vi "AudioTest.Result Table to CSV Measurements File.vi"(8 "error in":errorcluster, 9 "Results Table":T1[](array[typedef]) caption="Results", 10 "Test Name":string, 11 "UUT Dir":path) -> (0 "error out":errorcluster, 3 "Out File":path)   [LabVIEW 2018]
uses:
  Common/Utils/Results/Result.Results Table Record.ctl
  <vilib>/KATE/Files/File Utils.lvlib
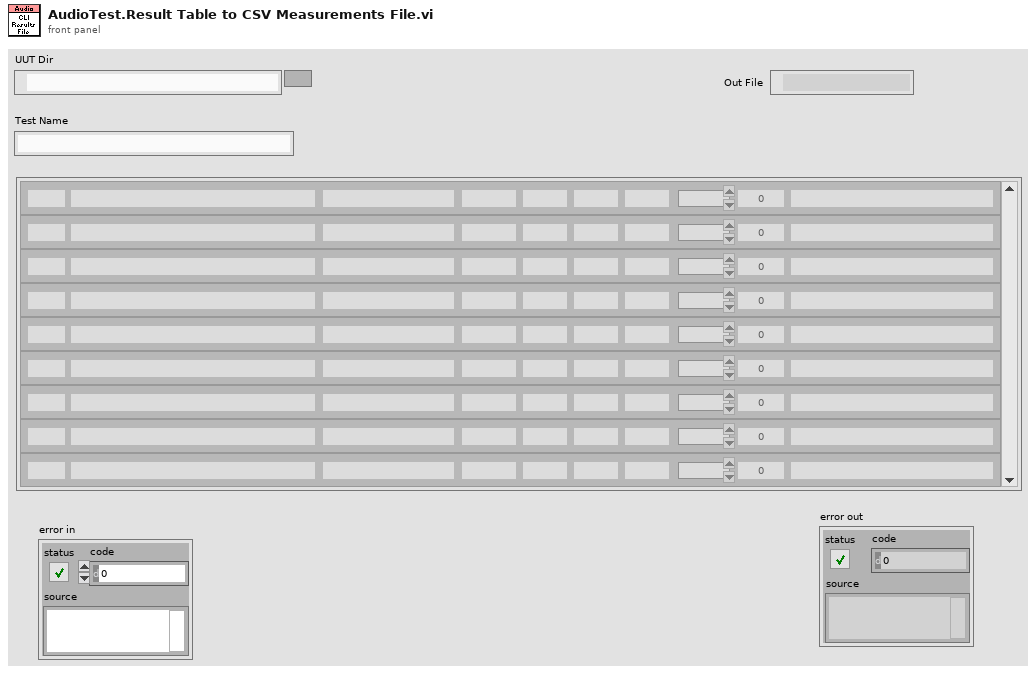
[diagram p1: front panel]
types:
  T1 = typedef "Result.Results Table Record.ctl" = cluster{"Cnt":i32, "Step":string, "Category":string, "Name":string, "Value":string, "Units":string, "LimType":string, "LL":string, "UL":string, "Status":string, "Status Color":u32, "Code":i32, "Desc":string}
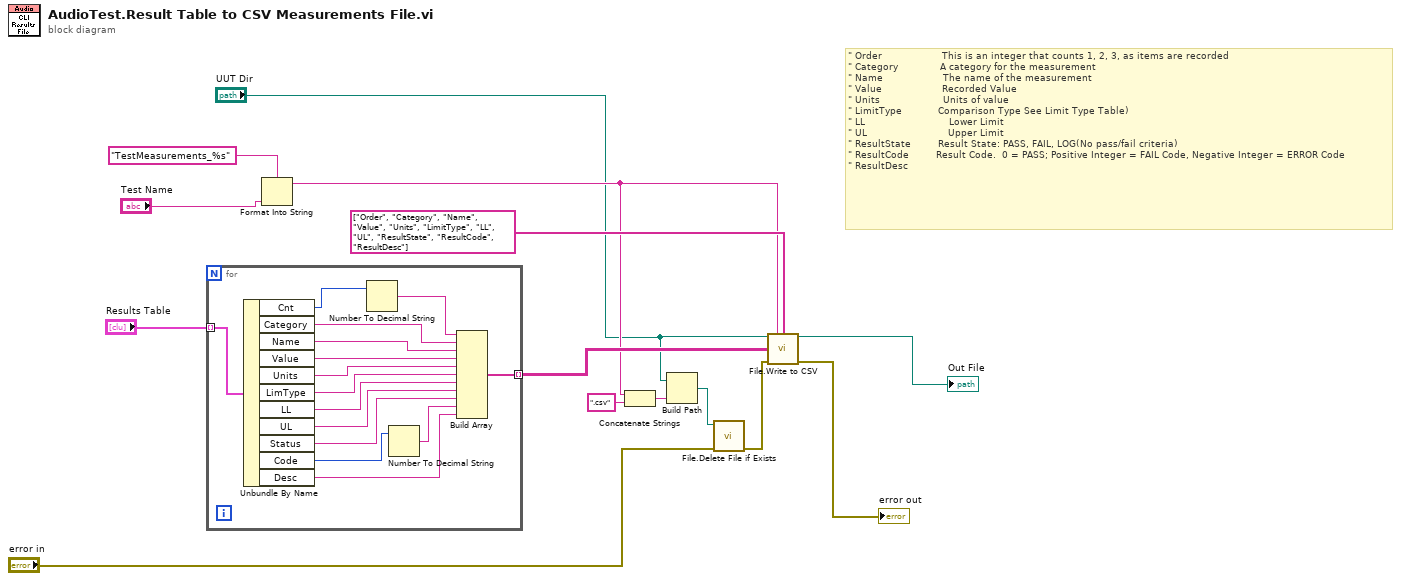
[diagram p0: block diagram]
diagram:
  # "\"\tOrder                    This is an integer that counts 1, 2, 3, as items are recorded\n\"\tCategory              A category for the measurement  \n\"\tName                    The name of the measurement\n\"\tValue                    Recorded Value\n\"\tUnits                     Units of value\n\"\tLimitType            Comparison Type See Limit Type Table) \n\"\tLL                            Lower Limit\n\"\tUL                           Upper Limit\n\"\tResultState         Result State: PASS, FAIL, LOG(No pass/fail criteria)\n\"\tResultCode         Result Code.  0 = PASS; Positive Integer = FAIL Code, Negative Integer = ERROR Code\n\"\tResultDesc"
  n1 = for {
    tunnel: "Results Table" -> [w29] mode=indexing
    tunnel: [w15] -> w10 mode=indexing
    n2 = Unbundle By Name(w29) -> ("Cnt"=w28:i32, "Category"=w25:string, "Name"=w24:string, "Value"=w23:string, "Units"=w22:string, "LimType"=w21:string, "LL"=w20:string, "UL"=w19:string, "Status"=w18:string, "Code"=w27:i32, "Desc"=w16:string)
    n3 = Number To Decimal String(number=w28) -> (decimal integer string=w26:string)  [unwired: 1 in]
    n4 = Number To Decimal String(number=w27) -> (decimal integer string=w17:string)  [unwired: 1 in]
    n5 = Build Array(w26, w25, w24, w23, w22, w21, w20, w19, w18, w17, w16) -> (w15:string[])
  }
  n6 = Format Into String(format string="TestMeasurements_%s", "Test Name") -> (resulting string=w6:string)  [unwired: 2 in, 1 out]
  n7 = Concatenate Strings(w6, ".csv" ("string")) -> (w5:string)
  n8 = Build Path(base path="UUT Dir", name or relative path=w5) -> (appended path=w1:path)
  n9 = call "File.Delete File if Exists.vi"("error in"="error in", "Path"=w1) -> ("error out"=w2:errorcluster)  [unwired: 8 in, 1 out]
  n10 = call <vilib>:"File.Write to CSV.vi"("Folder"="UUT Dir", "FileRootName"=w6, "Header"=string[] ["Order", "Category", "Name", "Value", "Units", "LimitType", "LL", "UL", "ResultState", "ResultCode", "ResultDesc"], "2D"=w10, "error in"=w2) -> ("File Path"=→"Out File":path, "error out"=→"error out":errorcluster)  [unwired: 9 in]
